vi "ParseDMMValue.vi"(5 "DMM Data":u8[](array[numeric])) -> (2 "Value":dbl)   [LabVIEW 2011]
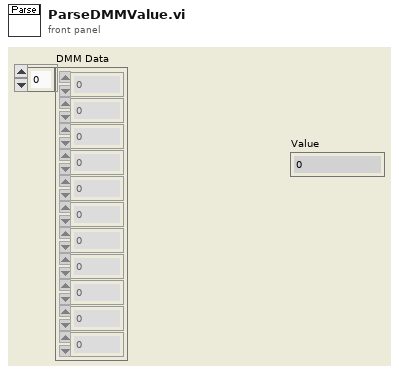
[diagram p1: front panel]
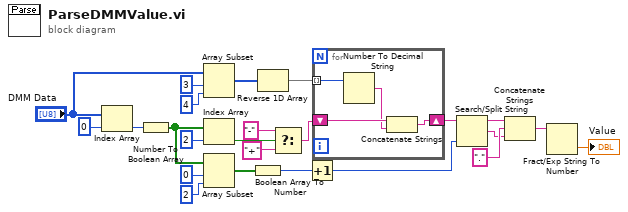
[diagram p0: block diagram]
diagram:
  n1 = Index Array(array="DMM Data", index=0) -> (element=w23:u8)
  n2 = Number To Boolean Array(number=w23) -> (Boolean array=w15:bool[])
  n3 = Array Subset(array="DMM Data", index=3, length=4) -> (w16:u8[])
  n4 = Index Array(array=w15, index=2) -> (element=w13:bool)
  n5 = Array Subset(array=w15, index=0, length=2) -> (w20:bool[])
  n6 = Boolean Array To Number(Boolean array=w20) -> (number=w7:u32)
  n7 = Reverse 1D Array(array=w16) -> (reversed array=w9:u8[])
  n8 = Select(t="-", s=w13, f="+") -> (s? t:f=w10:string)
  n9 = Increment(x=w7) -> (x+1=w3:u32)
  n10 = for {
    shift-right: [w27] -> w8
    shift-left: w10 -> [w26]
    tunnel: w9 -> [w28] mode=indexing
    n11 = Number To Decimal String(number=w28) -> (decimal integer string=w25:string)  [unwired: 1 out]
    n12 = Concatenate Strings(w26, w25) -> (w27:string)
  }
  n13 = Search/Split String(string=w8, offset (0)=w3) -> (substring before match=w6:string, match + rest of string=w4:string)  [unwired: 2 out]
  n14 = Concatenate Strings(w6, "." ("string"), w4) -> (w2:string)
  n15 = Fract/Exp String To Number(string=w2) -> (number=→"Value":dbl)  [unwired: 4 out]
